vi "mupGetExpr.vi"(8 "error in (no error)":errorcluster, 11 "muPar in":u64) -> (0 "error out":errorcluster, 2 "expr":string, 3 "muPar out":u64)   [LabVIEW 2015, in "mupLib.lvlib"]
doc: "Get the expression string"
uses:
  mupLib.lvlib
panel:
  # "Get the expression string"
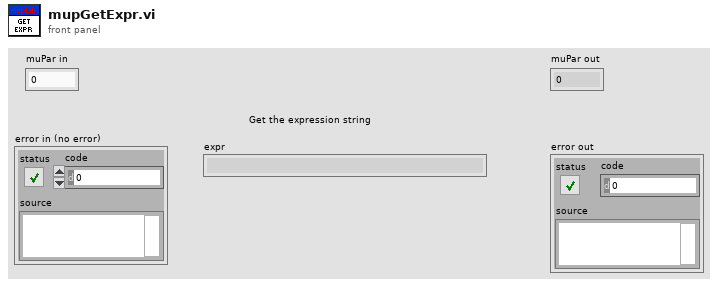
[diagram p1: front panel]
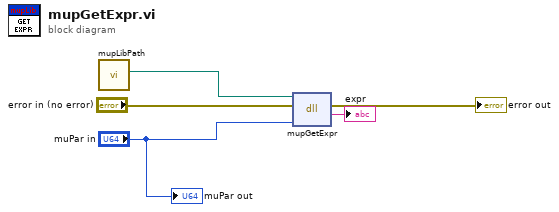
[diagram p0: block diagram]
diagram:
  n1 = call "mupLibPath.vi"() -> ("libmuparser path"=w4:path)  [unwired: 11 in]
  n2 = dll-call lib="C:/Program Files (x86)/National Instruments/LabVIEW 2015/resource/libmuparser-x32-lv.dll" fn="mupGetExpr"(path in=w4, error in="error in (no error)", "hParser"="muPar in") -> (error out=→"error out":errorcluster, "expr"=→"expr":string)  [unwired: 2 in, 1 out]
  "muPar out" <- "muPar in"
